vi "DSF.Engine.Pool.ID.Create.vi"(8 "error in (no error)":errorcluster, 10 "number of IDs":u32, 11 "ID Pool type":refnum<class "DSF.Engine.Pool.ID.lvclass">) -> (0 "error out":errorcluster, 3 "ID Pool out":refnum<class "DSF.Engine.Pool.ID.lvclass">)   [LabVIEW 2017, in "DSF.Engine.lvlib" / "DSF.Engine.Pool.ID.lvclass"]
uses:
  DSF.Engine.Pool.ID.lvclass
  C:/Git/DSF/Source/Engine/Classes/Thread Pool/DSF.Engine.Pool.lvclass
  DSF.Engine.Pool.lvclass
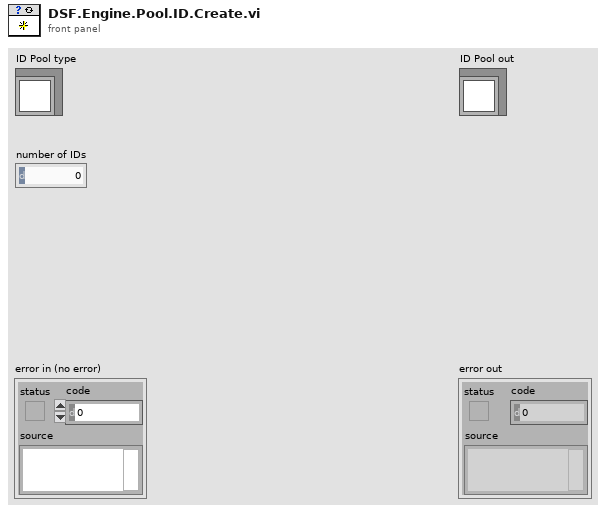
[diagram p1: front panel]
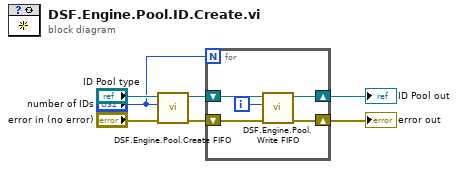
[diagram p0: block diagram]
diagram:
  n1 = call "DSF.Engine.Pool.Create FIFO.vi"("error in (no error)"="error in (no error)", "number of elements"="number of IDs", "Pool in"="ID Pool type") -> ("error out"=w4:errorcluster, "Pool out"=w5:refnum<class "DSF.Engine.Pool.ID.lvclass">)  [unwired: 7 in]
  n2 = for {
    N: "number of IDs" -> [_]
    shift-right: [w10] -> w3
    shift-left: w5 -> [w12]
    shift-right: [w9] -> w2
    shift-left: w4 -> [w11]
    i -> [w8]
    n3 = call "DSF.Engine.Pool.Write FIFO.vi"("error in (no error)"=w11, "element"=w8, "Pool in"=w12) -> ("error out"=w9:errorcluster, "Pool out"=w10:refnum<class "DSF.Engine.Pool.ID.lvclass">)  [unwired: 6 in, 1 out]
  }
  "error out" <- w2
  "ID Pool out" <- w3
